vi "MAINHARDWAREHDR_write.vi"(8 "error in (no error)":errorcluster, 10 "MAINHARDWAREHDR":T1, 11 "refnum in":refnum<file>) -> (0 "error out":errorcluster, 3 "refnum out":refnum<file>)   [LabVIEW 2012]
uses:
  TTTR_data_headers/MAINHARDWAREHDR.ctl
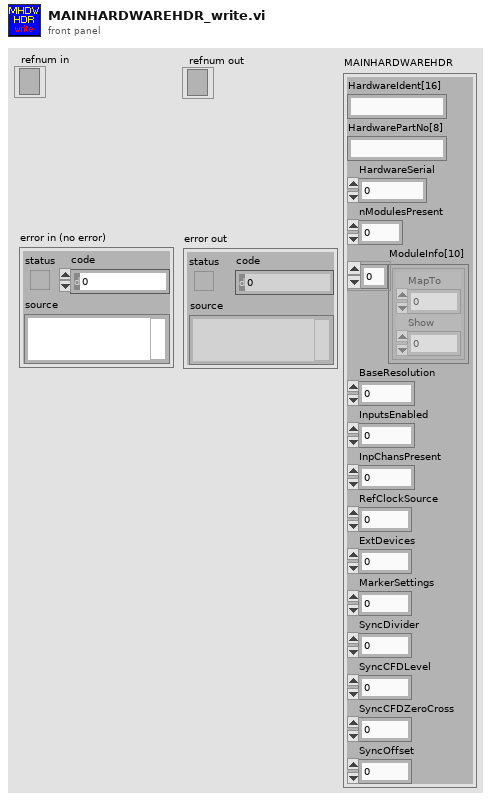
[diagram p1: front panel]
types:
  T1 = typedef "MAINHARDWAREHDR.ctl" = cluster{"HardwareIdent[16]":string, "HardwarePartNo[8]":string, "HardwareSerial":i32, "nModulesPresent":i32, "ModuleInfo[10]":cluster{"MapTo":i32, "Show":i32}[], "BaseResolution":dbl, "InputsEnabled":u64, "InpChansPresent":i32, "RefClockSource":i32, "ExtDevices":i32, "MarkerSettings":i32, "SyncDivider":i32, "SyncCFDLevel":i32, "SyncCFDZeroCross":i32, "SyncOffset":i32}
  T2 = enum16{"big-endian, network order", "native, host order", "little-endian"}
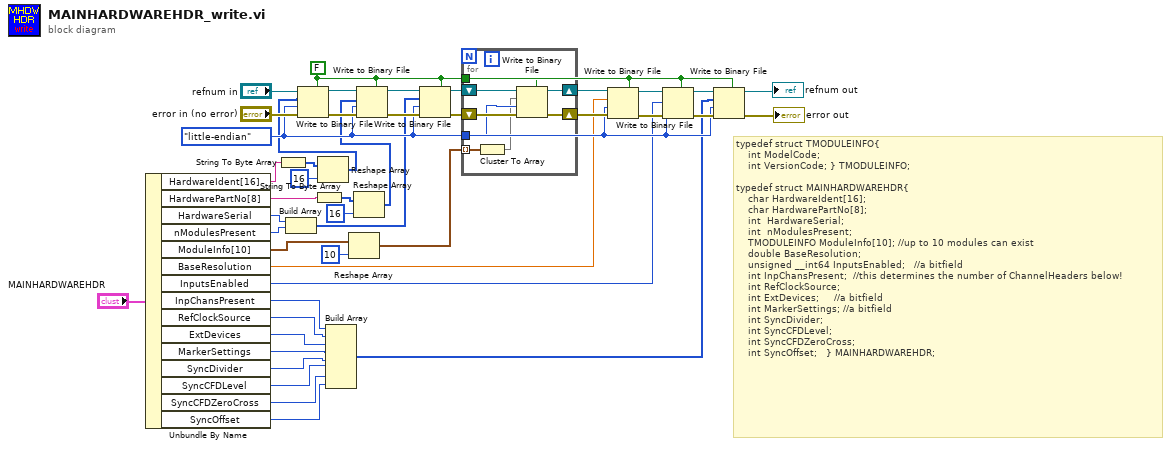
[diagram p0: block diagram]
diagram:
  w26 = FALSE ("prepend array or string size? (T)")
  w28 = T2."little-endian" ("byte order (0:big-endian, network order)")
  # "typedef\tstruct TMODULEINFO{\n\t\t\t\tint ModelCode;\n\t\t\t\tint VersionCode; } TMODULEINFO;\n\ntypedef struct MAINHARDWAREHDR{\t\t\n\t\t\t\tchar HardwareIdent[16];   \n\t\t\t\tchar HardwarePartNo[8]; \n\t\t\t\tint  HardwareSerial; \n\t\t\t\tint  nModulesPresent;     \n\t\t\t\tTMODULEINFO ModuleInfo[10]; //up to 10 modules can exist\n\t\t\t\tdouble BaseResolution;\n\t\t\t\tunsigned __int64 InputsEnabled;   //a bitfield\n\t\t\t\tint InpChansPresent;  //this determines the number of ChannelHeaders below!\n\t\t\t\tint RefClockSource;\n\t\t\t\tint ExtDevices;     //a bitfield\n\t\t\t\tint MarkerSettings; //a bitfield\n\t\t\t\tint SyncDivider;\n\t\t\t\tint SyncCFDLevel;\n\t\t\t\tint SyncCFDZeroCross;\n\t\t\t\tint SyncOffset;\t\t\t} MAINHARDWAREHDR;"
  n1 = Unbundle By Name("MAINHARDWAREHDR") -> ("HardwareIdent[16]"=w25:string, "HardwarePartNo[8]"=w19:string, "HardwareSerial"=w17:i32, "nModulesPresent"=w16:i32, "ModuleInfo[10]"=w14:cluster{"MapTo":i32, "Show":i32}[], "BaseResolution"=w11:dbl, "InputsEnabled"=w10:u64, "InpChansPresent"=w9:i32, "RefClockSource"=w8:i32, "ExtDevices"=w7:i32, "MarkerSettings"=w6:i32, "SyncDivider"=w5:i32, "SyncCFDLevel"=w4:i32, "SyncCFDZeroCross"=w3:i32, "SyncOffset"=w2:i32)
  n2 = String To Byte Array(string=w25) -> (unsigned byte array=w24:u8[])
  n3 = Build Array(w17, w16) -> (w15:i32[])
  n4 = String To Byte Array(string=w19) -> (unsigned byte array=w20:u8[])
  n5 = Reshape Array(w24, 16 ("dimension size")) -> (w22:u8[])
  n6 = Write to Binary File(file (use dialog)="refnum in", data=w22, error in="error in (no error)", 5:w26, 9:w28) -> (refnum out=w41:refnum<file>, error out=w42:errorcluster)  [unwired: 1 in, 1 out]
  n7 = Build Array(w9, w8, w7, w6, w5, w4, w3, w2) -> (w1:i32[])
  n8 = Reshape Array(w14, 10 ("dimension size")) -> (w12:cluster{"MapTo":i32, "Show":i32}[])
  n9 = Reshape Array(w20, 16 ("dimension size")) -> (w18:u8[])
  n10 = Write to Binary File(file (use dialog)=w41, data=w18, error in=w42, 5:w26, 9:w28) -> (refnum out=w39:refnum<file>, error out=w40:errorcluster)  [unwired: 1 in, 1 out]
  n11 = Write to Binary File(file (use dialog)=w39, data=w15, error in=w40, 5:w26, 9:w28) -> (refnum out=w37:refnum<file>, error out=w38:errorcluster)  [unwired: 1 in, 1 out]
  n12 = for {
    shift-right: [w49] -> w32
    shift-left: w38 -> [w52]
    shift-right: [w50] -> w30
    shift-left: w37 -> [w51]
    tunnel: w28 -> [w48]
    tunnel: w26 -> [w47]
    tunnel: w12 -> [w46] mode=indexing
    n13 = Cluster To Array(cluster=w46) -> (array=w45:i32[])
    n14 = Write to Binary File(file (use dialog)=w51, data=w45, error in=w52, 5:w47, 9:w48) -> (refnum out=w50:refnum<file>, error out=w49:errorcluster)  [unwired: 1 in, 1 out]
  }
  n15 = Write to Binary File(file (use dialog)=w30, data=w11, error in=w32, 5:w26, 9:w28) -> (refnum out=w29:refnum<file>, error out=w31:errorcluster)  [unwired: 1 in, 1 out]
  n16 = Write to Binary File(file (use dialog)=w29, data=w10, error in=w31, 5:w26, 9:w28) -> (refnum out=w35:refnum<file>, error out=w36:errorcluster)  [unwired: 1 in, 1 out]
  n17 = Write to Binary File(file (use dialog)=w35, data=w1, error in=w36, 5:w26, 9:w28) -> (refnum out=→"refnum out":refnum<file>, error out=→"error out":errorcluster)  [unwired: 1 in, 1 out]
